vi "Manage accounts.vi"(8 "error in":errorcluster, 10 "Users":T1[](array[typedef]), 11 "File action":T2) -> (0 "error out":errorcluster, 3 "Users":T1[](array[typedef]))   [LabVIEW 2015]
doc: "Read, write accounts data from/to txt file Accounts.txt."
uses:
  Controls/user.ctl
  Controls/File action.ctl
  <vilib>/Utility/file.llb/Read Delimited Spreadsheet (string).vi
  <vilib>/Utility/file.llb/Write Delimited Spreadsheet (string).vi
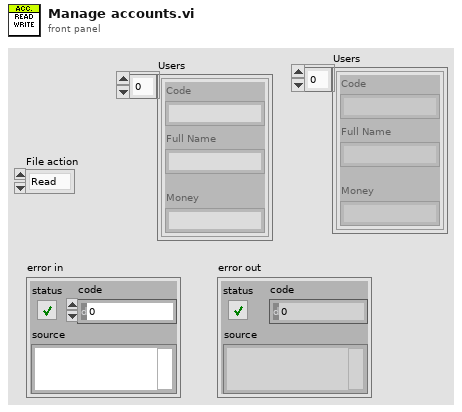
[diagram p1: front panel]
types:
  T1 = typedef "user.ctl" = cluster{"Code":string, "Full Name":string, "Money":string}
  T2 = typedef "File action.ctl" = enum16{"Read", "Write"}
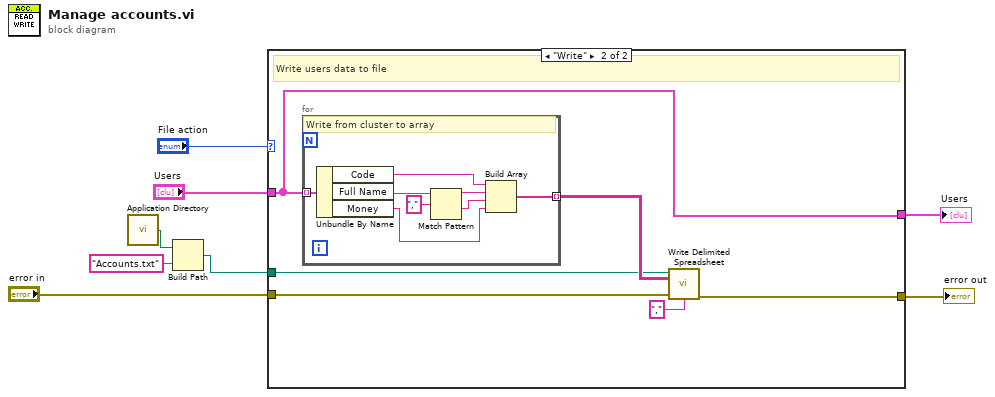
[diagram p0: block diagram]
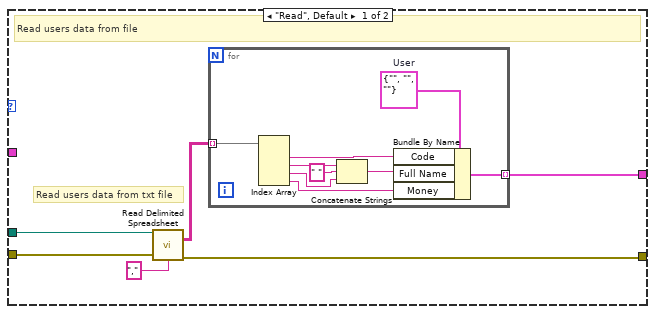
[diagram p2: hidden frame]
diagram:
  n1 = call <vilib>:"Application Directory.vi"() -> ("Application Directory"=w6:path)
  n2 = Build Path(base path=w6, name or relative path="Accounts.txt") -> (appended path=w8:path)
  n3 = case shown="\"Write\"" "File action" {
    tunnel: w8 -> [w14 w27]
    tunnel: "error in" -> [w13 w29]
    tunnel: "Users" -> [_ w25]
    tunnel: [w9 w26] -> w1
    tunnel: [w10 w25] -> w2
    frame "Read", Default {
      # "Read users data from txt file"
      # "Read users data from file"
      n4 = call-poly <vilib>:"Read Delimited Spreadsheet.vi"("file path (dialog if empty)"=w14, "error in (no error)"=w13, "delimiter (\\t)"="," ("delimiter (\\t)")) -> ("all rows"=w12:string[][], "error out"=w9:errorcluster)  [unwired: 7 in, 4 out]
      n5 = for {
        tunnel: w12 -> [w23] mode=indexing
        tunnel: [w15] -> w10 mode=indexing
        w19 = T1 {"Code"="", "Full Name"="", "Money"=""}  # User
        n6 = Index Array(array=w23) -> (element #1=w18:string, element #2=w22:string, element #3=w20:string, element #4=w16:string)  [unwired: 4 in]
        n7 = Concatenate Strings(w22, " " ("string"), w20) -> (w17:string)
        n8 = Bundle By Name(cluster=w19, "Code"=w18, "Full Name"=w17, "Money"=w16) -> (w15:T1)
      }
    }
    frame "Write" {
      # "Write users data to file"
      n9 = for {
        tunnel: w25 -> [w37] mode=indexing
        tunnel: [w30] -> w28 mode=indexing
        # "Write from cluster to array"
        n10 = Unbundle By Name(w37) -> ("Code"=w31:string, "Full Name"=w36:string, "Money"=w34:string)
        n11 = Match Pattern(string=w36, regular expression=",") -> (before substring=w32:string, after substring=w33:string)  [unwired: 1 in, 2 out]
        n12 = Build Array(w31, w32, w33, w34) -> (w30:string[])
      }
      n13 = call-poly <vilib>:"Write Delimited Spreadsheet.vi"("file path (dialog if empty)"=w27, "2D data"=w28, "error in (no error)"=w29, "delimiter (\\t)"="," ("delimiter (\\t)")) -> ("error out"=w26:errorcluster)  [unwired: 10 in, 1 out]
    }
  }
  "Users" <- w2
  "error out" <- w1
